vi "Shared Get Object Pointer.vi"(11 "Data in":refnum<class "Data.lvclass">) -> (1 "Object Pointer":i64, 2 "Assigned object pointer?":bool, 3 "Data out":refnum<class "Data.lvclass">)   [LabVIEW 2012, in "MDSplus.lvlib" / "Data.lvclass"]
uses:
  <vilib>/MDSplus/Classes/Data_Class/Data.lvclass
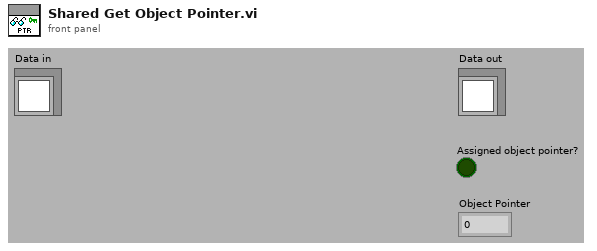
[diagram p1: front panel]
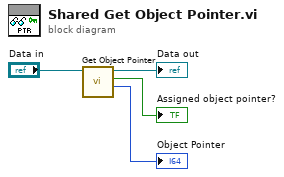
[diagram p0: block diagram]
diagram:
  n1 = call-dynamic "Get Object Pointer.vi"("Data in"="Data in") -> ("Object Pointer"=→"Object Pointer":i64, "Assigned object pointer?"=→"Assigned object pointer?":bool, "Data out"=→"Data out":refnum<class "Data.lvclass">)  [unwired: 8 in]
